vi "Configure Gamma Table.vi"(6 "Operation (0: Active Existing Table)":i32(ring) items=["Active Existing Table"=0, "Define Frequency Array"=1, "Rename Existing Table"=3, "Clear Existing Table"=4], 7 "New Table Name (\"MyTable\")":string="MyTable", 8 "error in (no error)":errorcluster, 9 "Table Data":i32[](array[numeric]), 10 "Gamma Table Name (\"DEFAULT\")":string="DEFAULT", 11 "VISA resource name":refnum<visa-resource-name>) -> (0 "error out":errorcluster, 3 "VISA resource name out":refnum<visa-resource-name>)   [LabVIEW 2014, in "Agilent U2000 Series.lvlib"]
doc: "Operates instrument for the gamma table functionality. Includes: Defines, Selects the gamma table to be used in the gamma correction, renames or clears specified gamma table. \n\nNote:\nThis VI is only applicable for U2040 X-Series."
uses:
  Agilent U2000 Series.lvlib
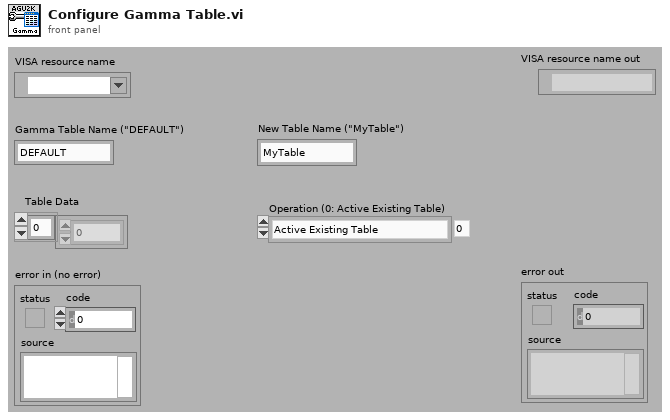
[diagram p1: front panel]
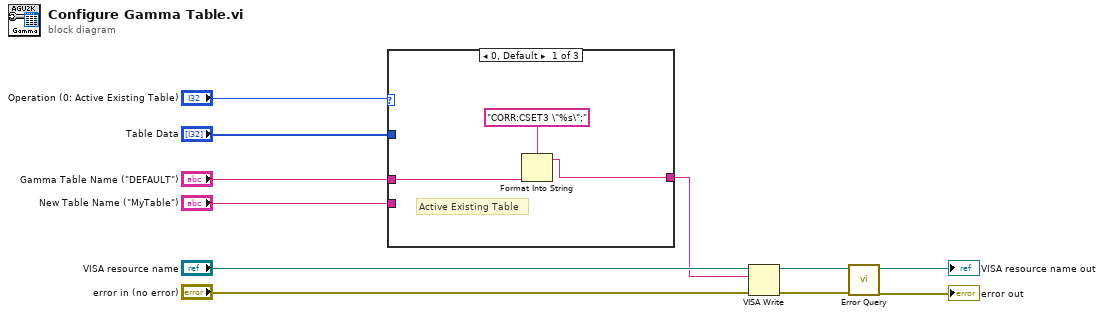
[diagram p0: block diagram]
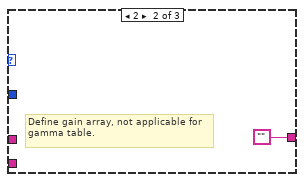
[diagram p2: hidden frame]
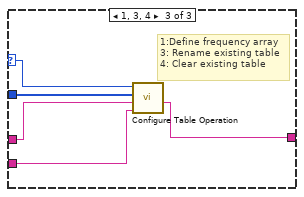
[diagram p3: hidden frame]
diagram:
  n1 = case shown="0, Default" "Operation (0: Active Existing Table)" {
    selector: "Operation (0: Active Existing Table)" -> [_ _ w20]
    tunnel: [w12 "" w17] -> w3
    tunnel: "Gamma Table Name (\"DEFAULT\")" -> [w14 _ w19]
    tunnel: "New Table Name (\"MyTable\")" -> [_ _ w18]
    tunnel: "Table Data" -> [_ _ w16]
    frame 0, Default {
      # "Active Existing Table"
      n2 = Format Into String(format string="CORR:CSET3 \"%s\";", w14) -> (resulting string=w12:string)  [unwired: 2 in, 1 out]
    }
    frame 2 {
      # "Define gain array, not applicable for gamma table."
    }
    frame 1, 3, 4 {
      # "1:Define frequency array\n3: Rename existing table\n4: Clear existing table"
      n3 = call "Configure Table Operation.vi"("New Table Name (\"MyTable\")"=w18, "Table Name (\"DEFAULT\")"=w19, "Table Data"=w16, "Operation (1: Define Frequency Array)"=w20) -> ("ResultString"=w17:string)  [unwired: 7 in]
    }
  }
  n4 = VISA Write(VISA resource name="VISA resource name", write buffer=w3, error in (no error)="error in (no error)") -> (VISA resource name out=w9:refnum<visa-resource-name>, error out=w8:errorcluster)  [unwired: 1 out]
  n5 = call "Error Query.vi"("error in (no error)"=w8, "VISA resource name"=w9) -> ("error out"=→"error out":errorcluster, "VISA resource name out"=→"VISA resource name out":refnum<visa-resource-name>)  [unwired: 6 in, 2 out]
